vi "7HP_Setup.vi"(2 "Analysis Info cluster In":T3[](array[typedef]) {"Sync Delay Time (s)" format="%.4f"; "Total Meas Time (s)" format="%_5g"; "Sd Error in Variance" format="%_3g"; "Skew_u" format="%_3g"; "% u'/U" format="%_3g"; "Sd Error in Mean" format="%_3g"; "Kurt_u" format="%_3g"; "u^4" format="%_3g"; "u^3" format="%_3g"; "U" format="%_3g"; "u^2" format="%_3g"}) -> (5 "Device port info":T1[](array[typedef]), 6 "Analysis Info cluster Out":T3[](array[typedef]) {"Sync Delay Time (s)" format="%.4f"; "Total Meas Time (s)" format="%_5g"; "Sd Error in Variance" format="%_3g"; "Skew_u" format="%_3g"; "% u'/U" format="%_3g"; "Sd Error in Mean" format="%_3g"; "Kurt_u" format="%_3g"; "u^4" format="%_3g"; "u^3" format="%_3g"; "U" format="%_3g"; "u^2" format="%_3g"}, 7 "7HP Info":T2(array[cluster]))   [LabVIEW 2022 SP3]
uses:
  Controls/Analysis_info_cluster.ctl
  Controls/Inst_type.ctl
  Controls/Instrument_Array.ctl
  Controls/channelState.ctl
  Acquisition/Device ID port info.ctl
  Globals/Meas_global.vi
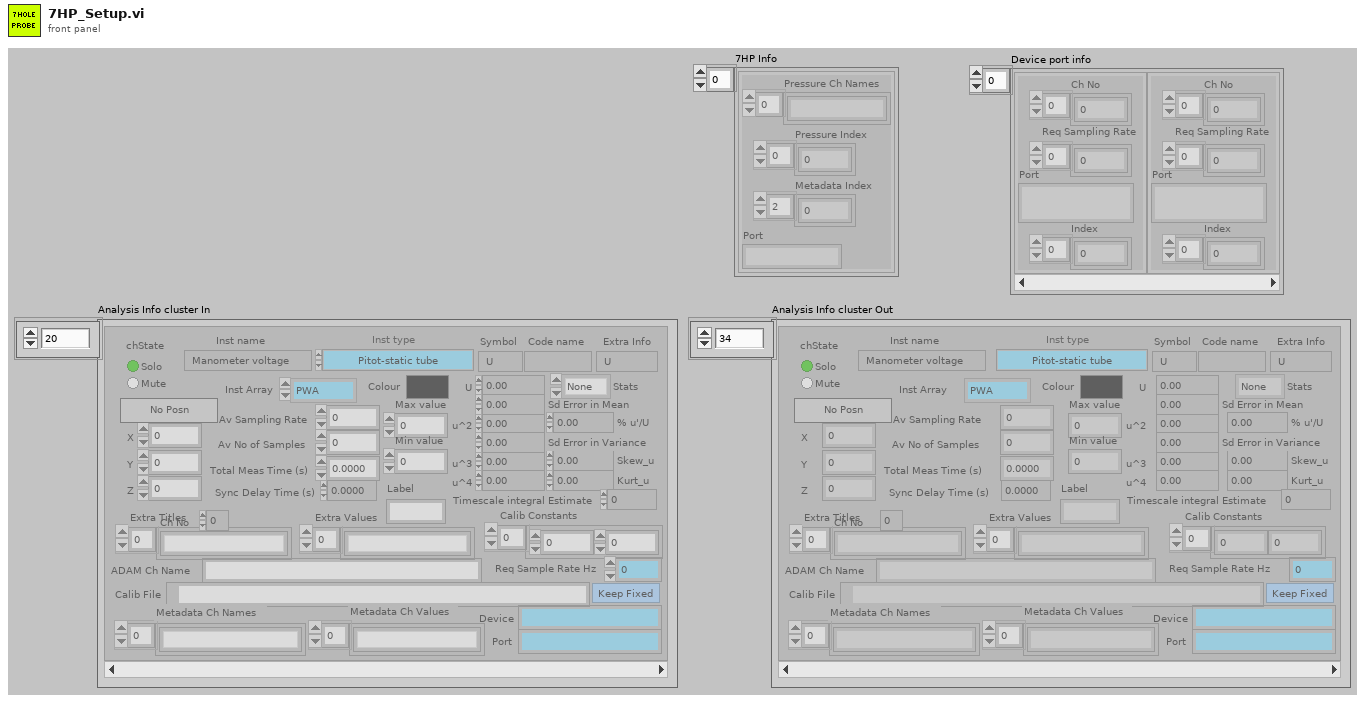
[diagram p1: front panel]
types:
  T1 = typedef "Device ID port info.ctl" = cluster{"Ch No":i16[], "Req Sampling Rate":dbl[], "Port":string, "Index":i32[]}
  T2 = cluster{"Pressure Ch Names":string[], "Pressure Index":i32[], "Metadata Index":i32[], "Port":string}[]
  T3 = typedef "Analysis_info_cluster.ctl" = cluster{"Colour":u32, "Inst type":T4, "Inst name":string, "Symbol":string, "Code name":string, "Extra Info":string, "Inst Array":T5, "Extra Titles":string[], "Extra Values":string[], "U":dbl, "u^2":dbl, "u^3":dbl, "u^4":dbl, "Skew_u":dbl, "Kurt_u":dbl, "Sd Error in Mean":dbl, "% u'/U":dbl, "X":dbl, "Y":dbl, "Z":dbl, "Timescale integral Estimate":dbl, "Sd Error in Variance":dbl, "Calib File":path, "Calib Constants":dbl[], "Output Position":bool, "Stats":enum16{"None", "Basic", "Full"}, "Av Sampling Rate":dbl, "Av No of Samples":dbl, "Total Meas Time (s)":dbl, "ADAM Ch Name":string, "Max value":dbl, "Min value":dbl, "Req Sample Rate Hz":dbl, "Sync Delay Time (s)":dbl, "Ch No":i16, "Device":string, "Use Latest Calib":bool, "Port":string, "Metadata Ch Names":string[], "Metadata Ch Values":string[], "Label":string, "chState":T6}
  T4 = typedef "Inst_type.ctl" = enum16{"Raw voltage", "Raw with zero offsetting", "Propeller anemometer", "Pressure Transducer", "Pitot-static tube", "Hot wire", "Cross wire 1", "Cross wire 2", "Generic Linear", "Generic Polynomial", "Generic BackPoly", "Fast FID", "Thermocouple", "Cold wire", "Pulsed Wire", "LDA Vel", "LDA Tran time", "LDA Arr time", "Microphone"}
  T5 = typedef "Instrument_Array.ctl" = enum16{"PWA", "LDA", "Analogue"}
  T6 = typedef "channelState.ctl" = enum32{"No Selection", "Solo", "Mute"}
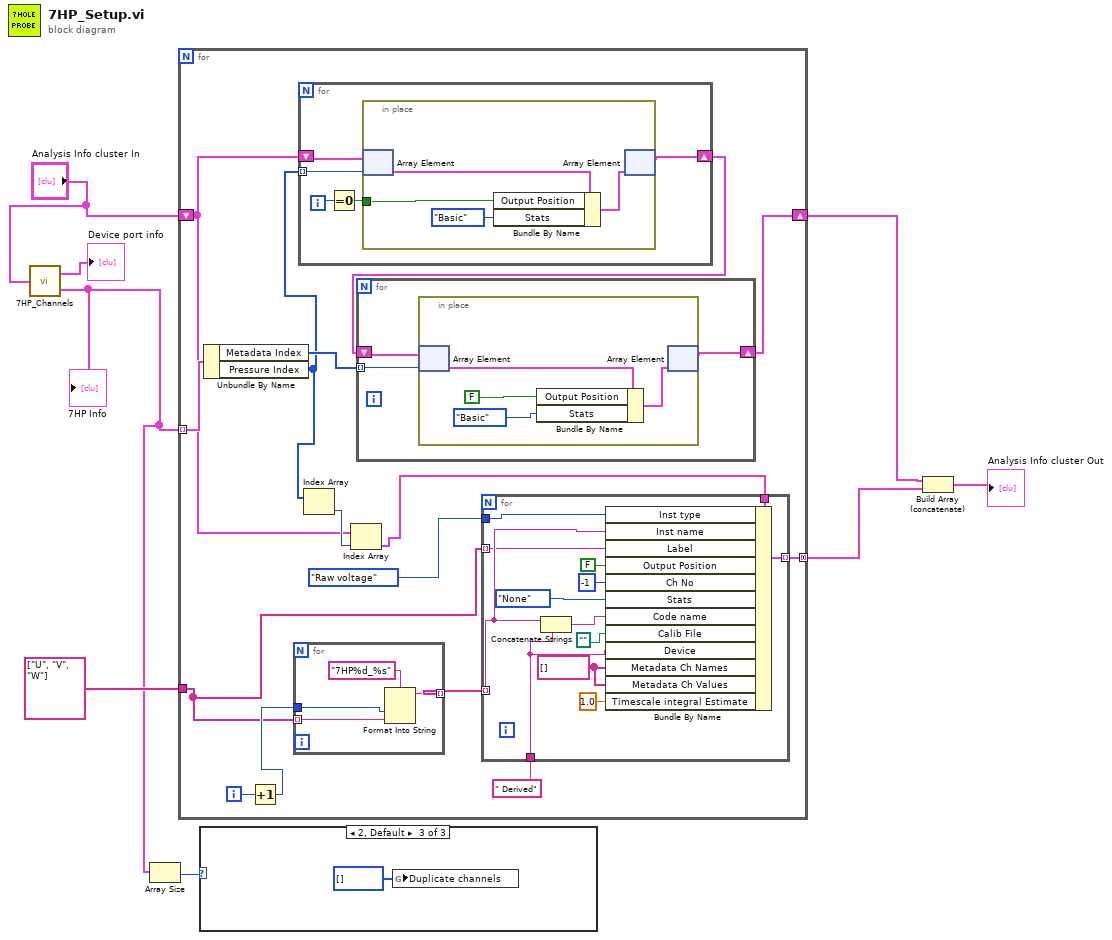
[diagram p0: block diagram]
diagram:
  n1 = call "7HP_Channels.vi"("Analysis Info cluster"="Analysis Info cluster In") -> ("Device port info"=→"Device port info":T1[], "7HP Info"=w3:T2)
  "7HP Info" <- w3
  n2 = Array Size(array=w3) -> (size(s)=w2:i32)
  n3 = for {
    tunnel: [w22] -> w8 mode=concatenating
    tunnel: string[] ["U", "V", "W"] ("appended array") -> [w9]
    tunnel: w3 -> [w16] mode=indexing
    shift-right: [w13] -> w4
    shift-left: "Analysis Info cluster In" -> [w15]
    i -> [w20]
    n4 = Unbundle By Name(w16) -> ("Metadata Index"=w12:i32[], "Pressure Index"=w10:i32[])
    n5 = Increment(x=w20) -> (x+1=w19:i32)
    n6 = for {
      tunnel: w9 -> [w40] mode=indexing
      tunnel: [w43] -> w21 mode=indexing
      tunnel: w19 -> [w42]
      n7 = Format Into String(format string="7HP%d_%s", w42, w40) -> (resulting string=w43:string)  [unwired: 2 in, 1 out]
    }
    n8 = for {
      shift-right: [w31] -> w14
      shift-left: w15 -> [w35]
      tunnel: w10 -> [w34] mode=indexing
      i -> [w33]
      n9 = Equal To 0?(x=w33) -> (x = 0?=w32:bool)
      n10 = in-place {
        in-place-border: w32 -> [w39]
        n11 = in-place-array #1(w35, w34) -> (w38:T3)
        n12 = Bundle By Name(cluster=w38, "Output Position"=w39, "Stats"=enum16{"None", "Basic", "Full"}."Basic") -> (w37:T3)
        n13 = in-place-array #1(w37) -> (w31:T3[])  [unwired: 1 out]
      }
    }
    n14 = Index Array(array=w10) -> (element=w18:i32)  [unwired: 1 in]
    n15 = Index Array(array=w15, index=w18) -> (element=w17:T3)
    n16 = for {
      shift-right: [w24] -> w13
      shift-left: w14 -> [w26]
      tunnel: w12 -> [w25] mode=indexing
      n17 = in-place {
        n18 = in-place-array #2(w26, w25) -> (w30:T3)
        n19 = Bundle By Name(cluster=w30, "Output Position"=FALSE ("Full Stats"), "Stats"=enum16{"None", "Basic", "Full"}."Basic") -> (w29:T3)
        n20 = in-place-array #2(w29) -> (w24:T3[])  [unwired: 1 out]
      }
    }
    n21 = for {
      tunnel: w17 -> [w56]
      tunnel: w21 -> [w51] mode=indexing
      tunnel: [w53] -> w22 mode=indexing
      tunnel: " Derived" -> [w48]
      tunnel: Inst_type."Raw voltage" ("Inst type") -> [w50]
      tunnel: w9 -> [w44] mode=indexing
      w47 = string[] [] ("Metadata Ch Names")
      n22 = Concatenate Strings(w51, w48) -> (w52:string)
      n23 = Bundle By Name(cluster=w56, "Inst type"=w50, "Inst name"=w51, "Label"=w44, "Output Position"=FALSE, "Ch No"=i16 -1, "Stats"=enum16{"None", "Basic", "Full"}."None", "Code name"=w52, "Calib File"=path "", "Device"=w48, "Metadata Ch Names"=w47, "Metadata Ch Values"=w47, "Timescale integral Estimate"=1.0) -> (w53:T3)
    }
  }
  n24 = case shown="2, Default" w2 {
    frame 0 {
    }
    frame 1 {
    }
    frame 2, Default {
      n25 = global write "Meas_global.vi" "Duplicate channels"(i32[] [] ("Duplicate channels")) -> ()
    }
  }
  n26 = Build Array (concatenate)(w4, w8) -> (→"Analysis Info cluster Out":T3[])
